vi "calcTravTime.vi"(7 "Mode":enum16{"Calc Vel & Acc", "Check Time"}(ring), 9 "Settings":T2, 11 "Total Distance":dbl[](array[numeric])) -> (0 "Channel Data":T1(array[cluster]), 1 "Accelerations":dbl[](array[numeric]), 3 "Velocities":dbl[](array[numeric]))   [LabVIEW 2017]
uses:
  Settings/Settings-Control.ctl
panel:
  out "Array":dbl[](array[numeric])
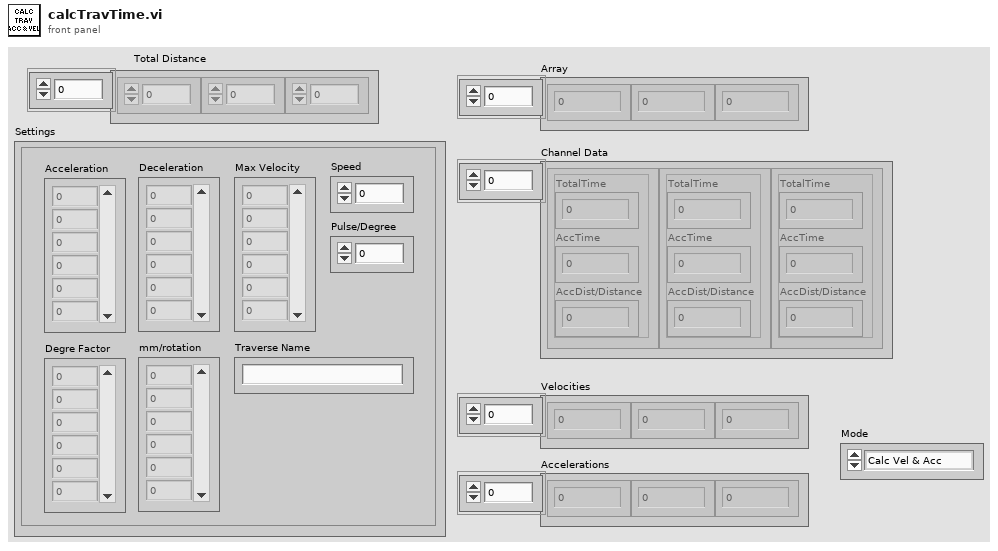
[diagram p1: front panel]
types:
  T1 = cluster{"TotalTime":dbl, "AccTime":dbl, "AccDist/Distance":dbl}[]
  T2 = typedef "Settings-Control.ctl" = cluster{"Acceleration":dbl[], "Deceleration":dbl[], "Max Velocity":dbl[], "Speed":dbl, "Pulse/Degree":dbl, "Degre Factor":dbl[], "mm/rotation":dbl[], "Traverse Name":string}
  T3 = cluster{"TotalTime":dbl, "AccTime":dbl, "AccDist/Distance":dbl}
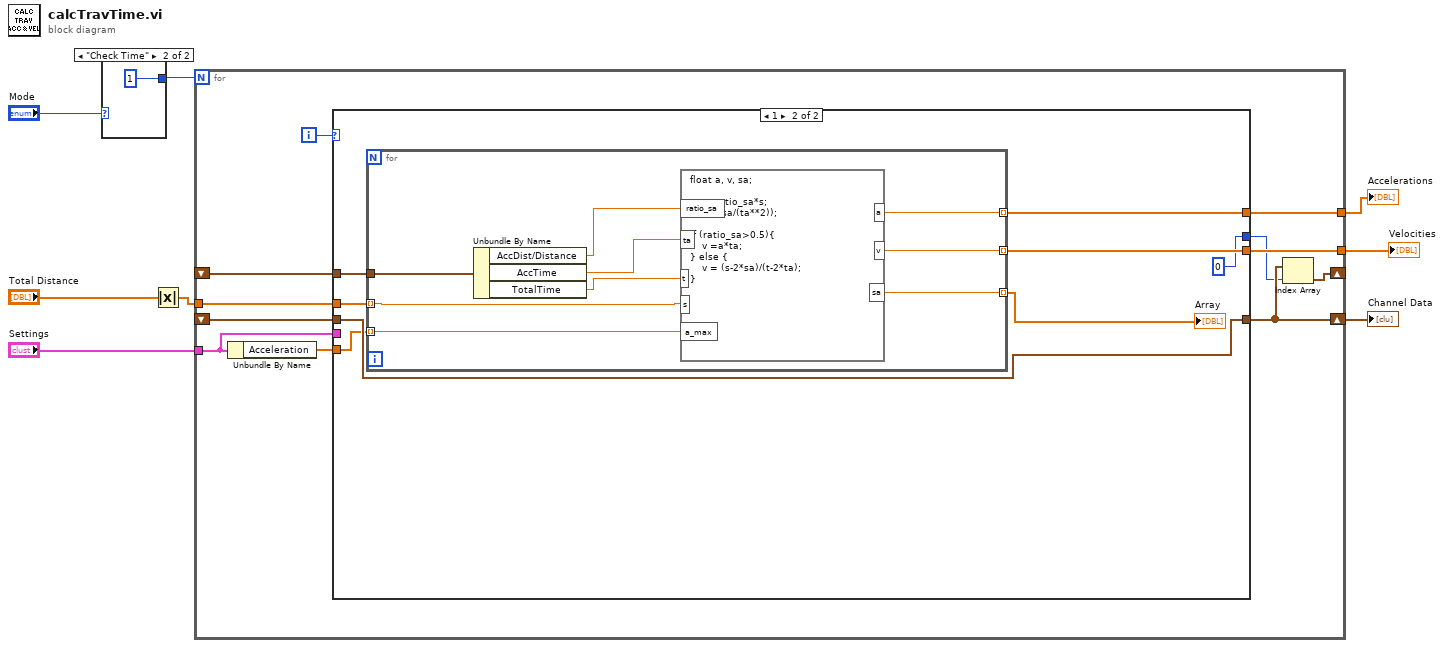
[diagram p0: block diagram]
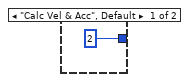
[diagram p2: hidden frame]
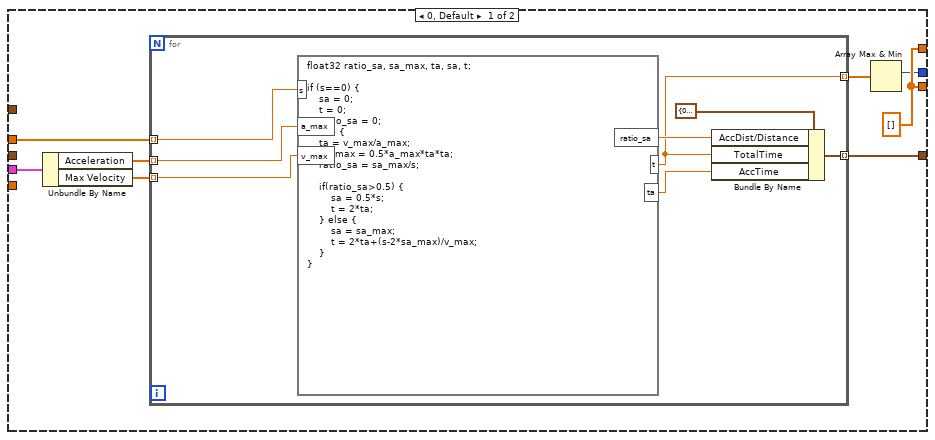
[diagram p3: hidden frame]
diagram:
  n1 = case shown="\"Check Time\"" "Mode" {
    tunnel: [2 1] -> w2
    frame "Calc Vel & Acc", Default {
    }
    frame "Check Time" {
    }
  }
  n2 = Absolute Value(x="Total Distance") -> (abs(x)=w6:dbl[])
  n3 = for {
    N: w2 -> [_]
    tunnel: "Settings" -> [w12]
    tunnel: w6 -> [w21]
    shift-right: [w13] -> _
    shift-left: _ -> [w19]
    tunnel: [w18] -> w5
    tunnel: [w17] -> w4
    shift-right: [w15] -> w1
    shift-left: _ -> [w16]
    i -> [w20]
    n4 = Unbundle By Name(w12) -> ("Acceleration"=w11:dbl[])
    n5 = case shown="1" w20 {
      tunnel: w12 -> [w29 _]
      tunnel: w21 -> [w25 w45]
      tunnel: w19 -> [_ w44]
      tunnel: [w24 w43] -> w18
      tunnel: [w24 w42] -> w17
      tunnel: [w23 w40] -> w15
      tunnel: w16 -> [_ w40]
      tunnel: [w22 0] -> w14
      tunnel: w11 -> [_ w38]
      frame 0, Default {
        w24 = dbl[] []
        n6 = Unbundle By Name(w29) -> ("Acceleration"=w28:dbl[], "Max Velocity"=w27:dbl[])
        n7 = for {
          tunnel: w28 -> [w37] mode=indexing
          tunnel: w27 -> [w36] mode=indexing
          tunnel: [w32] -> w23 mode=indexing
          tunnel: [w31] -> w26 mode=indexing
          tunnel: w25 -> [w30] mode=indexing
          n8 = formula code="float32 ratio_sa, sa_max, ta, sa, t;\n\nif (s==0) {\n    sa = 0;\n    t = 0;\n    ratio_sa = 0;\n} else {\n    ta = v_max/a_max;\n    sa_max = 0.5*a_max*ta*ta;\n    ratio_sa = sa_max/s;\n\n    if(ratio_sa>0.5) {\n        sa = 0.5*s;\n        t = 2*ta;\n    } else {\n        sa = sa_max;\n        t = 2*ta+(s-2*sa_max)/v_max;\n    }\n}"("s"=w30, "a_max"=w37, "v_max"=w36) -> ("ratio_sa"=w34:sgl, "t"=w31:sgl, "ta"=w33:sgl)
          n9 = Bundle By Name(cluster=T3 {"TotalTime"=0.0, "AccTime"=0.0, "AccDist/Distance"=0.0} ("Cluster"), "AccDist/Distance"=w34, "TotalTime"=w31, "AccTime"=w33) -> (w32:T3)
        }
        n10 = Array Max & Min(array=w26) -> (max index (indices)=w22:i32)  [unwired: 3 out]
      }
      frame 1 {
        n11 = for {
          tunnel: w45 -> [w54] mode=indexing
          tunnel: w44 -> [w47]
          tunnel: [w53] -> w43 mode=indexing
          tunnel: [w52] -> w42 mode=indexing
          tunnel: [w51] -> w41 mode=indexing
          tunnel: w38 -> [w46] mode=indexing
          n12 = Unbundle By Name(w47) -> ("AccDist/Distance"=w48:dbl, "AccTime"=w49:dbl, "TotalTime"=w50:dbl)
          n13 = formula code="float a, v, sa;\n\nsa = ratio_sa*s;\na =(2*sa/(ta**2));\n\nif (ratio_sa>0.5){\n    v =a*ta;\n} else {\n    v = (s-2*sa)/(t-2*ta);\n}"("ratio_sa"=w48, "ta"=w49, "t"=w50, "s"=w54, "a_max"=w46) -> ("a"=w53:dbl, "v"=w52:dbl, "sa"=w51:dbl)
        }
        "Array" <- w41
      }
    }
    n14 = Index Array(array=w15, index=w14) -> (element=w13:T3)
  }
  "Accelerations" <- w5
  "Velocities" <- w4
  "Channel Data" <- w1
